vi "Func-엑셀 데이터를 그래프로 출력.vi"() -> ()   [LabVIEW 2015]
uses:
  <vilib>/Math Plots/3D Math Plots/3D Surface/3D Surface XCtrl/3D Surface.xctl
  <vilib>/Math Plots/3D Math Plots/3D Surface/3D Surface Datatype/3D Surface Datatype.lvclass
  <vilib>/Math Plots/3D Math Plots/3D Surface/3D Surface Datatype/Public/Plot Helper (Vector).vi
panel:
  out "3D Surface":refnum<class "3D Plot Datatype.lvclass">[](xcontrol) caption="교정 데이터 3D 그래프"
  out "그래프2 Y편차":dbl=129.91 format="%#.6f"
  out "그래프1 Y편차":dbl=1.2835496700000002 format="%#.6f"
  in  "그래프 팔레트 보기":bool=TRUE
  in  "Y축 2":string="챔버인가온도(℃)\t챔버측정온도(℃)\t보드온도(℃)\n-36.563\t-36.49\t-18.927\n-36.647\t-36.53\t-19.012\n-36.73\t-36.6\t-19.101\n-36.813\t-36.65\t-19.183\n-36.897\t-36.69\t-19.261\n-36.98\t-36.74\t-19.346\n-37.063\t-36.77\t-19.434\n-37.147\t-36.81\t-19.512\n-37.23\t-36.84\t-19.587\n-37.313\t-36.87\t-19.675\n-37.397\t-36.9\t-19.751\n-37.48\t-36.95\t-19.827\n-37.563\t-36.98\t-19.916\n-37.647\t-37.02\t-19.982\n-37.73\t-37.05\t-20.076\n-37.813\t-37.08\t-20.151\n-37.897\t-37.11\t-20.23\n-37.98\t-37.15\t-20.306\n-38.063\t-37.18\t-20.387\n-38.147\t-37.23\t-20.462\n-38.23\t-37.27\t-20.538\n-38.313\t-37.31\t-20.615\n-38.397\t-37.33\t-20.683\n-38.48\t-37.37\t-20.754\n-38.563\t-37.41\t-20.829\n-38.647\t-37.45\t-20.905\n-38.73\t-37.48\t-20.986\n-38.813\t-37.51\t-21.051\n-38.897\t-37.55\t-21.134\n-38.98\t-37.57\t-21.207\n-39.063\t-37.6\t-21.268\n-39.147\t-37.64\t-21.341\n-39.23\t-37.69\t-21.42\n-39.313\t-37.72\t-21.484\n-39.397\t-37.77\t-21.561\n-39.48\t-37.79\t-21.629\n-39.563\t-37.83\t-21.7\n-39.647\t-37.85\t-21.759\n-39.73\t-37.89\t-21.834\n-39.813\t-37.93\t-21.896\n-39.897\t-37.97\t-21.967\n-39.98\t-38.01\t-22.041\n-40.063\t-38.05\t-22.107\n-40\t-38.08\t-22.171\n-40\t-38.08\t-22.175\n-40\t-38.08\t-22.184\n-40\t-38.08\t-22.189\n-40\t-38.09\t-22.195\n-40\t-38.09\t-22.205\n-40\t-38.1\t-22.21\n-40\t-38.1\t-22.214\n-40\t-38.11\t-22.218\n-40\t-38.11\t-22.224\n-40\t-38.11\t-22.23\n-40\t-38.12\t-22.237\n-40\t-38.12\t-22.242\n-40\t-38.13\t-22.25\n-40\t-38.13\t-22.264\n-40\t-38.13\t-22.27\n-40\t-38.14\t-22.276\n-40\t-38.14\t-22.284\n-40\t-38.15\t-22.289\n-40\t-38.16\t-22.294\n-40\t-38.16\t-22.298\n-40\t-38.16\t-22.303\n-40\t-38.16\t-22.309\n-40\t-38.16\t-22.319\n-40\t-38.16\t-22.325\n-40\t-38.16\t-22.33\n-40\t-38.17\t-22.34\n-40\t-38.17\t-22.346\n-40\t-38.18\t-22.35\n-40\t-38.18\t-22.356\n-40\t-38.18\t-22.359\n-40\t-38.19\t-22.367\n-40\t-38.19\t-22.371\n-40\t-38.19\t-22.376\n-40\t-38.19\t-22.384\n-40\t-38.2\t-22.392\n-40\t-38.2\t-22.4\n-40\t-38.2\t-22.405\n-40\t-38.2\t-22.41\n-40\t-38.21\t-22.416\n-40\t-38.21\t-22.423\n-40\t-38.21\t-22.431\n-40\t-38.22\t-22.434\n-40\t-38.22\t-22.438\n-40\t-38.22\t-22.451\n-40\t-38.23\t-22.456\n-40\t-38.23\t-22.458\n-40\t-38.24\t-22.468\n-40\t-38.24\t-22.479\n-40\t-38.24\t-22.484\n-40\t-38.24\t-22.489\n-40\t-38.24\t-22.496\n-40\t-38.24\t-22.504\n-40\t-38.24\t-22.511\n-40\t-38.24\t-22.515\n-40\t-38.25\t-22.523\n-40\t-38.25\t-22.53\n-40\t-38.25\t-22.537\n-40\t-38.26\t-22.544\n-40\t-38.26\t-22.551\n-40\t-38.26\t-22.557\n-40\t-38.26\t-22.569\n-40\t-38.27\t-22.573\n-40\t-38.27\t-22.579\n-40\t-38.28\t-22.582\n-40\t-38.28\t-22.591\n-40\t-38.29\t-22.597\n-40\t-38.29\t-22.605\n-40\t-38.3\t-22.614\n-40\t-38.31\t-22.617\n-40\t-38.31\t-22.623\n-40\t-38.31\t-22.631\n-40\t-38.31\t-22.636\n-40\t-38.31\t-22.639\n-40\t-38.31\t-22.645\n-40\t-38.32\t-22.651\n-40\t-38.32\t-22.662\n-40\t-38.33\t-22.669\n-40\t-38.33\t-22.671\n-40\t-38.33\t-22.682\n-40\t-38.33\t-22.686\n-40\t-38.34\t-22.693\n-40\t-38.34\t-22.7\n-40\t-38.35\t-22.703\n-40\t-38.36\t-22.712\n-40\t-38.36\t-22.72\n-40\t-38.36\t-22.726\n-40\t-38.37\t-22.732\n-40\t-38.37\t-22.735\n-40\t-38.37\t-22.739\n-40\t-38.38\t-22.744\n-40\t-38.38\t-22.752\n-40\t-38.38\t-22.759\n-40\t-38.38\t-22.763\n-40\t-38.38\t-22.774\n-40\t-38.39\t-22.782\n-40\t-38.39\t-22.788\n-40\t-38.4\t-22.792\n-40\t-38.4\t-22.795\n-40\t-38.41\t-22.802\n-40\t-38.41\t-22.811\n-40\t-38.42\t-22.814\n-40\t-38.42\t-22.822\n-40\t-38.42\t-22.831\n-40\t-38.42\t-22.838\n-40\t-38.43\t-22.842\n-40\t-38.43\t-22.852\n-40\t-38.43\t-22.857\n-40\t-38.44\t-22.86\n-40\t-38.44\t-22.872\n-40\t-38.44\t-22.877\n-40\t-38.44\t-22.886\n-40\t-38.45\t-22.892\n-40\t-38.46\t-22.9\n-40\t-38.46\t-22.903\n-40\t-38.46\t-22.911\n-40\t-38.46\t-22.915\n-40\t-38.47\t-22.919\n-40\t-38.47\t-22.926\n-40\t-38.47\t-22.925\n-40\t-38.48\t-22.935\n-40\t-38.48\t-22.939\n-40\t-38.49\t-22.944\n-40\t-38.49\t-22.951\n-40\t-38.5\t-22.955\n-40\t-38.5\t-22.966\n-40\t-38.51\t-22.972\n-40\t-38.51\t-22.98\n-40\t-38.52\t-22.989\n-40\t-38.52\t-22.992\n-40\t-38.53\t-23.005\n-40\t-38.53\t-23.011\n-40\t-38.54\t-23.015\n-40\t-38.54\t-23.023\n-40\t-38.54\t-23.027\n-40\t-38.54\t-23.035\n-40\t-38.54\t-23.04\n-40\t-38.55\t-23.043\n-40\t-38.55\t-23.048\n-40\t-38.56\t-23.055\n-40\t-38.56\t-23.062\n-40\t-38.57\t-23.066\n-40\t-38.57\t-23.076\n-40\t-38.58\t-23.082\n-40\t-38.58\t-23.089\n-40\t-38.59\t-23.096\n-40\t-38.59\t-23.104\n-40\t-38.6\t-23.109\n-40\t-38.61\t-23.113\n-40\t-38.61\t-23.119\n-40\t-38.61\t-23.123\n-40\t-38.61\t-23.131\n-40\t-38.61\t-23.133\n-40\t-38.61\t-23.14\n-40\t-38.62\t-23.148\n-40\t-38.62\t-23.154\n-40\t-38.62\t-23.159\n-40\t-38.63\t-23.166\n-40\t-38.64\t-23.173\n-40\t-38.64\t-23.179\n-40\t-38.65\t-23.186\n-40\t-38.66\t-23.19\n-40\t-38.66\t-23.199\n-40\t-38.67\t-23.205\n-40\t-38.67\t-23.211\n-40\t-38.67\t-23.216\n-40\t-38.67\t-23.22\n-40\t-38.68\t-23.227\n-40\t-38.68\t-23.236\n-40\t-38.68\t-23.241\n-40\t-38.68\t-23.245\n-40\t-38.68\t-23.253\n-40\t-38.68\t-23.259\n-40\t-38.68\t-23.263\n-40\t-38.68\t-23.271\n-40\t-38.68\t-23.277\n-40\t-38.68\t-23.282\n-40\t-38.69\t-23.291\n-40\t-38.69\t-23.296\n-40\t-38.7\t-23.305\n-40\t-38.7\t-23.31\n-40\t-38.71\t-23.313\n-40\t-38.72\t-23.32\n-40\t-38.72\t-23.325\n-40\t-38.72\t-23.329\n-40\t-38.73\t-23.335\n-40\t-38.73\t-23.341\n-40\t-38.73\t-23.346\n-40\t-38.74\t-23.349\n-40\t-38.74\t-23.357\n-40\t-38.74\t-23.361\n-40\t-38.75\t-23.364\n-40\t-38.75\t-23.372\n-40\t-38.75\t-23.381\n-40\t-38.75\t-23.391\n-40\t-38.75\t-23.398\n-40\t-38.75\t-23.406\n-40\t-38.76\t-23.413\n-40\t-38.76\t-23.42\n-40\t-38.76\t-23.42\n-40\t-38.77\t-23.424\n-40\t-38.77\t-23.43\n-40\t-38.77\t-23.436\n-40\t-38.78\t-23.441\n-40\t-38.78\t-23.45\n-40\t-38.79\t-23.459\n-40\t-38.79\t-23.466\n-40\t-38.8\t-23.472\n-40\t-38.8\t-23.473\n-40\t-38.8\t-23.477\n-40\t-38.81\t-23.484\n-40\t-38.81\t-23.492\n-40\t-38.82\t-23.497\n-40\t-38.82\t-23.505\n-40\t-38.83\t-23.511\n-40\t-38.83\t-23.519\n-40\t-38.83\t-23.527\n-40\t-38.84\t-23.529\n-40\t-38.84\t-23.532\n-40\t-38.85\t-23.54\n-40\t-38.85\t-23.55\n-40\t-38.86\t-23.552\n-40\t-38.86\t-23.557\n-40\t-38.86\t-23.561\n-40\t-38.87\t-23.567\n-40\t-38.87\t-23.573\n-40\t-38.88\t-23.575\n-40\t-38.88\t-23.582\n-40\t-38.89\t-23.589\n-40\t-38.89\t-23.599\n-40\t-38.89\t-23.6\n-40\t-38.9\t-23.605\n-40\t-38.9\t-23.611\n-40\t-38.9\t-23.614\n-40\t-38.9\t-23.621\n-40\t-38.9\t-23.626\n-40\t-38.91\t-23.635\n-40\t-38.91\t-23.642\n-40\t-38.92\t-23.646\n-40\t-38.92\t-23.653\n-40\t-38.92\t-23.662\n-40\t-38.93\t-23.666\n-40\t-38.93\t-23.67\n-40\t-38.93\t-23.675\n-40\t-38.94\t-23.683\n-40\t-38.94\t-23.686\n-40\t-38.95\t-23.69\n-40\t-38.95\t-23.696\n-40\t-38.96\t-23.703\n-40\t-38.96\t-23.713\n-40\t-38.97\t-23.718\n-40\t-38.97\t-23.725\n-40\t-38.97\t-23.732\n-40\t-38.98\t-23.732\n-40\t-38.98\t-23.737\n-40\t-38.98\t-23.741\n-40\t-38.99\t-23.746\n-40\t-38.99\t-23.75\n-40\t-38.99\t-23.756\n-40\t-38.99\t-23.763\n-40\t-38.99\t-23.77\n-40\t-38.99\t-23.776\n-40\t-39\t-23.781\n-40\t-39\t-23.787\n-40\t-39\t-23.796\n-40\t-39.01\t-23.804\n-40\t-39.01\t-23.809\n-40\t-39.02\t-23.818\n-40\t-39.03\t-23.826\n-40\t-39.03\t-23.832\n-40\t-39.04\t-23.839\n-40\t-39.04\t-23.841\n-40\t-39.04\t-23.846\n-40\t-39.05\t-23.852\n-40\t-39.05\t-23.852\n-40\t-39.06\t-23.857\n-40\t-39.06\t-23.866\n-40\t-39.06\t-23.873\n-40\t-39.06\t-23.875\n-40\t-39.07\t-23.879\n-40\t-39.07\t-23.888\n-40\t-39.08\t-23.893\n-40\t-39.08\t-23.896\n-40\t-39.08\t-23.907\n-40\t-39.09\t-23.918\n-40\t-39.09\t-23.927\n-40\t-39.1\t-23.931\n-40\t-39.1\t-23.936\n-40\t-39.11\t-23.945\n-40\t-39.12\t-23.945\n-40\t-39.12\t-23.947\n-40\t-39.13\t-23.953\n-40\t-39.13\t-23.959\n-40\t-39.13\t-23.965\n-40\t-39.13\t-23.971\n-40\t-39.13\t-23.973\n-40\t-39.13\t-23.978\n-40\t-39.13\t-23.988\n-40\t-39.14\t-23.993\n-40\t-39.14\t-23.995\n-40\t-39.15\t-24.003\n-40\t-39.15\t-24.01\n-40\t-39.16\t-24.016\n-40\t-39.16\t-24.018\n-40\t-39.17\t-24.023\n-40\t-39.17\t-24.025\n-40\t-39.17\t-24.032\n-40\t-39.17\t-24.037\n-40\t-39.18\t-24.041\n-40\t-39.18\t-24.048\n-40\t-39.19\t-24.05\n-40\t-39.19\t-24.059\n-40\t-39.2\t-24.064\n-40\t-39.2\t-24.069\n-40\t-39.2\t-24.075\n-40\t-39.2\t-24.085\n-40\t-39.2\t-24.094\n-40\t-39.21\t-24.101\n-40\t-39.21\t-24.109\n-40\t-39.22\t-24.113\n-40\t-39.22\t-24.116\n-40\t-39.22\t-24.122\n-40\t-39.23\t-24.127\n-40\t-39.23\t-24.13\n-40\t-39.23\t-24.136\n-40\t-39.24\t-24.144\n-40\t-39.24\t-24.151\n-40\t-39.25\t-24.156\n-40\t-39.25\t-24.159\n-40\t-39.25\t-24.165\n-40\t-39.26\t-24.17\n-40\t-39.26\t-24.172\n-40\t-39.27\t-24.174\n-40\t-39.27\t-24.179\n-40\t-39.28\t-24.186\n-40\t-39.28\t-24.191\n-40\t-39.28\t-24.199\n-40\t-39.29\t-24.205\n-40\t-39.29\t-24.213\n-40\t-39.29\t-24.219\n-40\t-39.29\t-24.222\n-40\t-39.3\t-24.228\n-40\t-39.3\t-24.236\n-40\t-39.3\t-24.241\n-40\t-39.31\t-24.248\n-40\t-39.31\t-24.255\n-40\t-39.32\t-24.262\n-40\t-39.32\t-24.268\n-40\t-39.33\t-24.274\n-40\t-39.33\t-24.28\n-40\t-39.34\t-24.281\n-40\t-39.34\t-24.293\n-40\t-39.35\t-24.3\n-40\t-39.35\t-24.304\n-40\t-39.35\t-24.304\n-40\t-39.35\t-24.308\n-40\t-39.35\t-24.313\n-40\t-39.36\t-24.32\n-40\t-39.36\t-24.325\n-40\t-39.37\t-24.33\n-40\t-39.37\t-24.34\n-40\t-39.37\t-24.347\n-40\t-39.37\t-24.355\n-40\t-39.38\t-24.357\n-40\t-39.38\t-24.363\n-40\t-39.39\t-24.366\n-40\t-39.39\t-24.376\n-40\t-39.4\t-24.377\n-40\t-39.4\t-24.379\n-40\t-39.41\t-24.388\n-40\t-39.41\t-24.395\n-40\t-39.42\t-24.4\n-40\t-39.42\t-24.405\n-40\t-39.43\t-24.411\n-40\t-39.43\t-24.415\n-40\t-39.43\t-24.423\n-40\t-39.43\t-24.423\n-40\t-39.43\t-24.43\n-40\t-39.43\t-24.436\n-40\t-39.44\t-24.442\n-40\t-39.44\t-24.447\n-40\t-39.44\t-24.457\n-40\t-39.44\t-24.462\n-40\t-39.44\t-24.468\n-40\t-39.45\t-24.475\n-40\t-39.45\t-24.481\n-40\t-39.46\t-24.488\n-40\t-39.46\t-24.491\n-40\t-39.47\t-24.497\n-40\t-39.47\t-24.499\n-40\t-39.47\t-24.505\n-40\t-39.47\t-24.511\n-40\t-39.48\t-24.515\n-40\t-39.48\t-24.52\n-40\t-39.49\t-24.525\n-40\t-39.49\t-24.529\n-40\t-39.49\t-24.535\n-40\t-39.49\t-24.54\n-40\t-39.49\t-24.545\n-40\t-39.5\t-24.549\n-40\t-39.5\t-24.555\n-40\t-39.5\t-24.566\n-40\t-39.5\t-24.571\n-40\t-39.5\t-24.572\n-40\t-39.5\t-24.577\n-40\t-39.51\t-24.586\n-40\t-39.51\t-24.591\n-40\t-39.51\t-24.593\n-40\t-39.52\t-24.596\n-40\t-39.52\t-24.605\n-40\t-39.53\t-24.609\n-40\t-39.53\t-24.614\n-40\t-39.53\t-24.618\n-40\t-39.54\t-24.627\n-40\t-39.54\t-24.631\n-40\t-39.54\t-24.633\n-40\t-39.55\t-24.643\n-40\t-39.55\t-24.647\n-40\t-39.56\t-24.65\n-40\t-39.56\t-24.654\n-40\t-39.57\t-24.663\n-40\t-39.57\t-24.669\n-40\t-39.58\t-24.675\n-40\t-39.58\t-24.681\n-40\t-39.58\t-24.688\n-40\t-39.58\t-24.689\n-40\t-39.59\t-24.698\n-40\t-39.59\t-24.702\n-40\t-39.59\t-24.706\n-40\t-39.6\t-24.712\n-40\t-39.61\t-24.718\n-40\t-39.61\t-24.73\n-40\t-39.62\t-24.735\n-40\t-39.62\t-24.739\n-40\t-39.62\t-24.74\n-40\t-39.63\t-24.743\n-40\t-39.63\t-24.745\n-40\t-39.63\t-24.748\n-40\t-39.63\t-24.749\n-40\t-39.63\t-24.755\n-40\t-39.64\t-24.763\n-40\t-39.64\t-24.772\n-40\t-39.64\t-24.78\n-40\t-39.65\t-24.786\n-40\t-39.65\t-24.793\n-40\t-39.65\t-24.799\n-40\t-39.65\t-24.807\n-40\t-39.65\t-24.814\n-40\t-39.66\t-24.817\n-40\t-39.66\t-24.823\n-40\t-39.66\t-24.827\n-40\t-39.66\t-24.834\n-40\t-39.67\t-24.837\n-40\t-39.67\t-24.839\n-40\t-39.68\t-24.843\n-40\t-39.68\t-24.848\n-40\t-39.68\t-24.855\n-40\t-39.68\t-24.86\n-40\t-39.69\t-24.865\n-40\t-39.69\t-24.873\n-40\t-39.69\t-24.873\n-40\t-39.7\t-24.877\n-40\t-39.7\t-24.879\n-40\t-39.7\t-24.881\n-40\t-39.7\t-24.886\n-40\t-39.7\t-24.891\n-40\t-39.7\t-24.898\n-40\t-39.71\t-24.903\n-40\t-39.71\t-24.911\n-40\t-39.71\t-24.916\n-40\t-39.71\t-24.92\n-40\t-39.71\t-24.929\n-40\t-39.71\t-24.937\n-40\t-39.72\t-24.94\n-40\t-39.72\t-24.952\n-40\t-39.72\t-24.96\n-40\t-39.73\t-24.967\n-40\t-39.73\t-24.975\n-40\t-39.73\t-24.977\n-40\t-39.73\t-24.984\n-40\t-39.73\t-24.985\n-40\t-39.73\t-24.985\n-40\t-39.73\t-24.989\n-40\t-39.74\t-24.995\n-40\t-39.74\t-25.001\n-40\t-39.74\t-25.004\n-40\t-39.74\t-25.01\n-40\t-39.74\t-25.017\n-40\t-39.75\t-25.022\n-40\t-39.75\t-25.025\n-40\t-39.75\t-25.03\n-40\t-39.75\t-25.037\n-40\t-39.76\t-25.043\n-40\t-39.76\t-25.047\n-40\t-39.76\t-25.05\n-40\t-39.76\t-25.058\n-40\t-39.77\t-25.06\n-40\t-39.77\t-25.061\n-40\t-39.77\t-25.067\n-40\t-39.77\t-25.07\n-40\t-39.78\t-25.076\n-40\t-39.78\t-25.08\n-40\t-39.79\t-25.087\n-40\t-39.79\t-25.094\n-40\t-39.8\t-25.099\n-40\t-39.8\t-25.105\n-40\t-39.8\t-25.106\n-40\t-39.8\t-25.115\n-40\t-39.8\t-25.119\n-40\t-39.81\t-25.125\n-40\t-39.81\t-25.134\n-40\t-39.81\t-25.139\n-40\t-39.81\t-25.147\n-40\t-39.81\t-25.148\n-40\t-39.81\t-25.153\n-40\t-39.82\t-25.159\n-40\t-39.82\t-25.166\n-40\t-39.82\t-25.17\n-40\t-39.83\t-25.175\n-40\t-39.83\t-25.18\n-40\t-39.83\t-25.185\n-40\t-39.83\t-25.186\n-40\t-39.84\t-25.19\n-40\t-39.84\t-25.193\n-40\t-39.84\t-25.195\n-40\t-39.84\t-25.204\n-40\t-39.84\t-25.208\n-40\t-39.85\t-25.211\n-40\t-39.85\t-25.216\n-40\t-39.85\t-25.221\n-40\t-39.86\t-25.225\n-40\t-39.86\t-25.231\n-40\t-39.87\t-25.237\n-40\t-39.87\t-25.243\n-40\t-39.87\t-25.252\n-40\t-39.88\t-25.256\n-40\t-39.88\t-25.263\n-40\t-39.88\t-25.268\n-40\t-39.88\t-25.271\n-40\t-39.88\t-25.279\n-40\t-39.88\t-25.28\n-40\t-39.88\t-25.286\n-40\t-39.88\t-25.291\n-40\t-39.88\t-25.299\n-40\t-39.88\t-25.303\n-40\t-39.88\t-25.307\n-40\t-39.89\t-25.312\n-40\t-39.9\t-25.318\n-40\t-39.91\t-25.319\n-40\t-39.92\t-25.323\n-40\t-39.93\t-25.328\n-40\t-39.94\t-25.335\n-40\t-39.95\t-25.341\n-40\t-39.96\t-25.346\n-40\t-39.97\t-25.352\n-40\t-39.98\t-25.358\n-40\t-39.99\t-25.364\n-40\t-40\t-25.37\n-40\t-39.98\t-25.373\n-40\t-39.98\t-25.375\n-40\t-39.98\t-25.379\n-40\t-39.98\t-25.387\n-40\t-39.98\t-25.389\n-40\t-39.98\t-25.396\n-40\t-39.98\t-25.402\n-40\t-39.98\t-25.407\n-40\t-39.98\t-25.417\n-40\t-39.98\t-25.42\n-40\t-39.98\t-25.425\n-40\t-39.98\t-25.43\n-40\t-39.98\t-25.435\n-40\t-39.99\t-25.442\n-40\t-39.99\t-25.444\n-40\t-39.99\t-25.447\n-40\t-39.99\t-25.453\n-40\t-39.99\t-25.459\n-40\t-39.99\t-25.462\n-40\t-39.99\t-25.466\n-40\t-39.99\t-25.47\n-40\t-39.99\t-25.472\n-40\t-39.99\t-25.476\n-40\t-39.99\t-25.48\n-40\t-39.99\t-25.485\n-40\t-39.99\t-25.487\n-40\t-39.99\t-25.498\n-40\t-39.99\t-25.506\n-40\t-39.99\t-25.511\n-40\t-39.99\t-25.518\n-40\t-39.99\t-25.525\n-40\t-39.99\t-25.531\n-40\t-39.99\t-25.534\n-40\t-39.99\t-25.54\n-40\t-39.99\t-25.542\n-40\t-39.99\t-25.55\n-40\t-39.99\t-25.555\n-40\t-39.99\t-25.559\n-40\t-39.99\t-25.565\n-40\t-39.99\t-25.569\n-40\t-39.99\t-25.574\n-40\t-39.99\t-25.579\n-40\t-39.99\t-25.579\n-40\t-39.99\t-25.583\n-40\t-39.99\t-25.591\n-40\t-39.99\t-25.593\n-40\t-39.99\t-25.598\n-40\t-39.99\t-25.603\n-40\t-39.99\t-25.61\n-40\t-39.99\t-25.616\n-40\t-39.99\t-25.62\n-40\t-39.99\t-25.63\n-40\t-39.99\t-25.636\n-40\t-39.99\t-25.643\n-40\t-39.99\t-25.65\n-40\t-39.99\t-25.655\n-40\t-39.99\t-25.664\n-40\t-39.99\t-25.663\n-40\t-39.99\t-25.668\n-40\t-39.99\t-25.674\n-40\t-39.99\t-25.675\n-40\t-39.99\t-25.676\n-40\t-39.99\t-25.683\n-40\t-39.99\t-25.69\n-40\t-39.99\t-25.694\n-40\t-39.99\t-25.7\n-40\t-39.99\t-25.704\n-40\t-39.99\t-25.707\n-40\t-39.99\t-25.711\n-40\t-39.99\t-25.714\n-40\t-39.99\t-25.716\n-40\t-40\t-25.726\n-40\t-40\t-25.73\n-40\t-40\t-25.736\n-40\t-40\t-25.742\n-40\t-40\t-25.745\n-40\t-40\t-25.751\n-40\t-40\t-25.75\n-40\t-40\t-25.755\n-40\t-40\t-25.763\n-40\t-40\t-25.771\n-40\t-40\t-25.777\n-40\t-40\t-25.78\n-40\t-40\t-25.787\n-40\t-40\t-25.792\n-40\t-40\t-25.794\n-40\t-40\t-25.8\n-40\t-40\t-25.806\n-40\t-40\t-25.817\n-40\t-40\t-25.821\n-40\t-40\t-25.824\n-40\t-40\t-25.826\n-40\t-40\t-25.832\n-40\t-40\t-25.834\n-40\t-40\t-25.832\n-40\t-39.99\t-25.841\n-40\t-40\t-25.848\n-40\t-40\t-25.854\n-40\t-40\t-25.855\n-40\t-39.99\t-25.859\n-40\t-40\t-25.864\n-40\t-40\t-25.866\n-40\t-40\t-25.869\n-40\t-40\t-25.871\n-40\t-40\t-25.879\n-40\t-40\t-25.885\n-40\t-40\t-25.891\n-40\t-40\t-25.898\n-40\t-40\t-25.902\n-40\t-40\t-25.908\n-40\t-40\t-25.911\n-40\t-40\t-25.916\n-40\t-40\t-25.922\n-40\t-40\t-25.922\n-40\t-40\t-25.925\n-40\t-40\t-25.929\n-40\t-40\t-25.936\n-40\t-40\t-25.94\n-40\t-40\t-25.945\n-40\t-40\t-25.955\n-40\t-40\t-25.961\n-40\t-40\t-25.969\n-40\t-40\t-25.975\n-40\t-40\t-25.977\n-40\t-40\t-25.982\n-40\t-40\t-25.986\n-40\t-40\t-25.985\n-40\t-40\t-25.987\n-40\t-40\t-25.993\n-40\t-40\t-25.998\n-40\t-40\t-26.001\n-40\t-40\t-26.005\n-40\t-40\t-26.016\n-40\t-40\t-26.02\n-40\t-40\t-26.02\n-40\t-40\t-26.02\n-40\t-40\t-26.027\n-40\t-40\t-26.03\n-40\t-40\t-26.035\n-40\t-40\t-26.043\n-40\t-40\t-26.046\n-40\t-40\t-26.052\n-40\t-40\t-26.055\n-40\t-40\t-26.06\n-40\t-40\t-26.062\n-40\t-40\t-26.071\n-40\t-40\t-26.079\n-40\t-40\t-26.086\n-40\t-40\t-26.091\n-40\t-40\t-26.095\n-40\t-40\t-26.1\n-40\t-40\t-26.101\n-40\t-40\t-26.102\n-40\t-40\t-26.103\n-40\t-40\t-26.112\n-40\t-40\t-26.116\n-40\t-40\t-26.122\n-40\t-40\t-26.13\n-40\t-40\t-26.136\n-40\t-40\t-26.144\n-40\t-40\t-26.147\n-40\t-40\t-26.15\n-40\t-40\t-26.154\n-40\t-40\t-26.156\n-40\t-40\t-26.163\n-40\t-40\t-26.164\n-40\t-40\t-26.173\n-40\t-40\t-26.176\n-40\t-40\t-26.179\n-40\t-40\t-26.183\n-40\t-40\t-26.188\n-40\t-40\t-26.192\n-40\t-40\t-26.195\n-40\t-40\t-26.2\n-40\t-40\t-26.204\n-40\t-40\t-26.211\n-40\t-40\t-26.213\n-40\t-40\t-26.215\n-40\t-40\t-26.22\n-40\t-40\t-26.224\n-40\t-40\t-26.23\n-40\t-40\t-26.235\n-40\t-40\t-26.239\n-40\t-40\t-26.246\n-40\t-40\t-26.252\n-40\t-40\t-26.26\n-40\t-40\t-26.262\n-40\t-40\t-26.268\n-40\t-40\t-26.271\n-40\t-40\t-26.274\n-40\t-40\t-26.279\n-40\t-40\t-26.279\n-40\t-40\t-26.282\n-40\t-40\t-26.289\n-40\t-40\t-26.291\n-40\t-40\t-26.293\n-40\t-40\t-26.297\n-40\t-40\t-26.305\n-40\t-40\t-26.313\n-40\t-40\t-26.318\n-40\t-40\t-26.321\n-40\t-40\t-26.326\n-40\t-40\t-26.331\n-40\t-40\t-26.33\n-40\t-40\t-26.333\n-40\t-40\t-26.337\n-40\t-40\t-26.343\n-40\t-40\t-26.35\n-40\t-40\t-26.352\n-40\t-40\t-26.359\n-40\t-40\t-26.364\n-40\t-40\t-26.37\n-40\t-40\t-26.371\n-40\t-40\t-26.38\n-40\t-40\t-26.385\n-40\t-40\t-26.389\n-40\t-40\t-26.394\n-40\t-40\t-26.396\n-40\t-40\t-26.4\n-40\t-40\t-26.403\n-40\t-40\t-26.41\n-40\t-40\t-26.415\n-40\t-40.02\t-26.417\n-40\t-40.02\t-26.421\n-40\t-40.02\t-26.425\n-40\t-40.02\t-26.428\n-40\t-40.02\t-26.432\n-40\t-40.02\t-26.436\n-40\t-40.02\t-26.44\n-40\t-40.02\t-26.443\n-40\t-40.02\t-26.449\n-40\t-40.02\t-26.454\n-40\t-40.02\t-26.454\n-40\t-40.02\t-26.457\n-40\t-40.02\t-26.465\n-40\t-40.02\t-26.471\n-40\t-40.02\t-26.476\n-40\t-40.02\t-26.484\n-40\t-40.02\t-26.488\n-40\t-40.02\t-26.493\n-40\t-40.02\t-26.498\n-40\t-40.02\t-26.501\n-40\t-40.02\t-26.503\n-40\t-40.02\t-26.506\n-40\t-40.02\t-26.513\n-40\t-40.02\t-26.517\n-40\t-40.02\t-26.523\n-40\t-40.02\t-26.527\n-40\t-40.02\t-26.528\n-40\t-40.02\t-26.532\n-40\t-40.02\t-26.534\n-40\t-40.02\t-26.535\n-40\t-40.02\t-26.54\n-40\t-40.02\t-26.545\n-40\t-40.02\t-26.552\n-40\t-40.02\t-26.558\n-40\t-40.02\t-26.565\n-40\t-40.02\t-26.571\n-40\t-40.02\t-26.579\n-40\t-40.02\t-26.58\n-40\t-40.02\t-26.583\n-40\t-40.02\t-26.586\n-40\t-40.02\t-26.59\n-40\t-40.02\t-26.594\n-40\t-40.02\t-26.595\n-40\t-40.02\t-26.597\n-40\t-40.02\t-26.602\n-40\t-40.02\t-26.609\n-40\t-40.02\t-26.611\n-40\t-40.02\t-26.615\n-40\t-40.02\t-26.62\n-40\t-40.02\t-26.627\n-40\t-40.02\t-26.63\n-40\t-40.02\t-26.634\n-40\t-40.02\t-26.635\n-40\t-40.02\t-26.638\n-40\t-40.02\t-26.646\n-40\t-40.02\t-26.649\n-40\t-40.02\t-26.652\n-40\t-40.02\t-26.657\n-40\t-40.02\t-26.664\n-40\t-40.02\t-26.668\n-40\t-40.02\t-26.67\n-40\t-40.02\t-26.673\n-40\t-40.02\t-26.679\n-40\t-40.02\t-26.684\n-40\t-40.02\t-26.691\n-40\t-40.02\t-26.689\n-40\t-40.02\t-26.695\n-40\t-40.02\t-26.7\n-40\t-40.02\t-26.702\n-40\t-40.02\t-26.707\n-40\t-40.02\t-26.708\n-40\t-40.02\t-26.716\n-40\t-40.02\t-26.721\n-40\t-40.02\t-26.721\n-40\t-40.02\t-26.725\n-40\t-40.02\t-26.729\n-40\t-40.02\t-26.732\n-40\t-40.02\t-26.733\n-40\t-40.02\t-26.738\n-40\t-40.02\t-26.743\n-40\t-40.02\t-26.746\n-40\t-40.02\t-26.752\n-40\t-40.02\t-26.757\n-40\t-40.02\t-26.763\n-40\t-40.02\t-26.765\n-40\t-40.02\t-26.767\n-40\t-40.02\t-26.77\n-40\t-40.02\t-26.775\n-40\t-40.02\t-26.778\n-40\t-40.02\t-26.78\n-40\t-40.02\t-26.786\n-40\t-40.02\t-26.791\n-40\t-40.02\t-26.796\n-40\t-40.02\t-26.805\n-40\t-40.02\t-26.81\n-40\t-40.02\t-26.818\n-40\t-40.02\t-26.823\n-40\t-40.02\t-26.826\n-40\t-40.02\t-26.828\n-40\t-40.02\t-26.829\n-40\t-40.02\t-26.83\n-40\t-40.02\t-26.828\n-40\t-40.02\t-26.835\n-40\t-40.02\t-26.839\n-40\t-40.02\t-26.843\n-40\t-40.02\t-26.847\n
